vi "Obtain Notifier.vi"(8 "error in (no error)":errorcluster, 11 "CVT_DBL in":refnum<class "CVT_DBL.lvclass">) -> (0 "error out":errorcluster, 3 "CVT_DBL out":refnum<class "CVT_DBL.lvclass">)   [LabVIEW 2024, in "Current Value Table.lvlib" / "CVT_DBL.lvclass"]
uses:
  CVT_DBL.lvclass
  CVT_DBL.lvclass/CVT_DBL.ctl
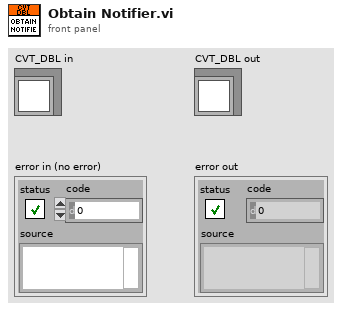
[diagram p1: front panel]
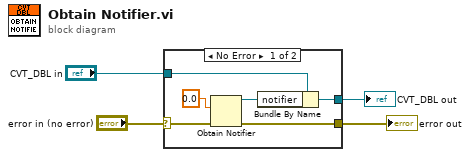
[diagram p0: block diagram]
diagram:
  n1 = case shown="No Error" "error in (no error)" {
    selector: "error in (no error)" -> [w8 w12]
    tunnel: [w7 w12] -> w3
    tunnel: [w6 w11] -> w1
    tunnel: "CVT_DBL in" -> [w10 w11]
    frame No Error {
      n2 = Obtain Notifier(notification data type=0.0 ("element data type"), error in (no error)=w8) -> (notifier out=w9:refnum<notifier>, error out=w7:errorcluster)  [unwired: 2 in, 1 out]
      n3 = Bundle By Name(cluster=w10, "notifier"=w9) -> (w6:refnum<class "CVT_DBL.lvclass">)
    }
    frame Error {
    }
  }
  "error out" <- w3
  "CVT_DBL out" <- w1
